vi "MissionLocation.vi"(8 "Error In":errorcluster, 11 "PassBouy in":refnum<class "PassBouy.lvclass">) -> (0 "Error Out":errorcluster, 2 "element":T1 {"North" format="%#_10f"; "East" format="%#_8f"}, 3 "PassBouy out":refnum<class "PassBouy.lvclass">)   [LabVIEW 2013, in "PassBouy.lvclass"]
doc: "Get the location of this mission for maps and such. In this case, it's the midpoint between the two buoys to be passed through."
uses:
  PassBouy.lvclass
  Data/TypeDefs/UTM Location.ctl
  GenericMission/GenericMission.lvclass
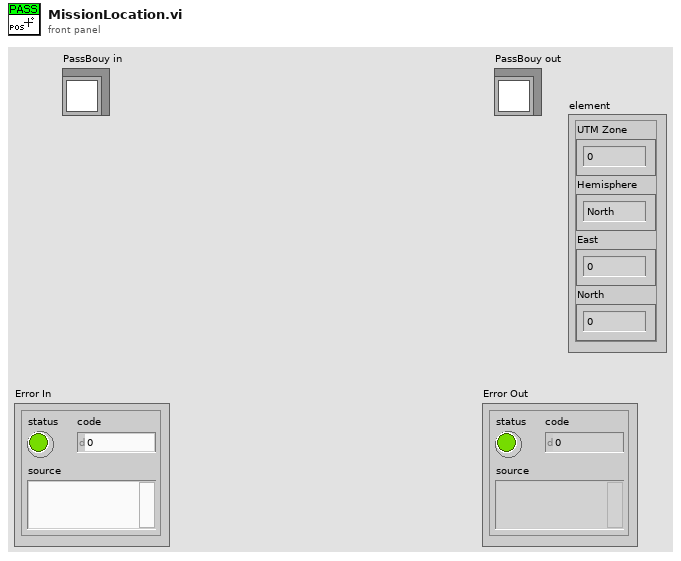
[diagram p1: front panel]
types:
  T1 = typedef "UTM Location.ctl" = cluster{"UTM Zone":dbl, "Hemisphere":enum16{"North", "South"}, "East":dbl, "North":dbl}
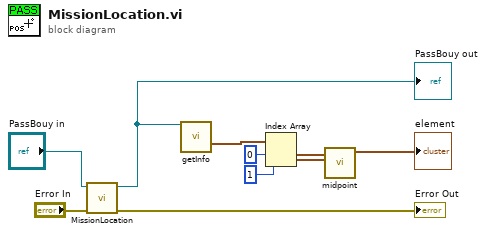
[diagram p0: block diagram]
diagram:
  n1 = call-parent "MissionLocation.vi"("Error In"="Error In", "GenericMission in"="PassBouy in") -> ("Error Out"=→"Error Out":errorcluster, "GenericMission out"=w1:refnum<class "PassBouy.lvclass">)  [unwired: 7 in, 1 out]
  "PassBouy out" <- w1
  n2 = call-dynamic "getInfo.vi"("GenericMission in"=w1) -> ("Points of Interest"=w2:T1[])  [unwired: 6 in, 8 out]
  n3 = Index Array(array=w2, index #1=0 ("index"), index #2=1 ("index")) -> (element #1=w5:T1, element #2=w4:T1)
  n4 = call "midpoint.vi"("UTM Location 2"=w4, "UTM Location"=w5) -> ("UTM Location 3"=→"element":T1)  [unwired: 8 in, 1 out]
